vi "sub_new amplitude to array.vi"(6 "Index Row":i32, 7 "All Random Array In":fxp<+/-,32,16>[][](array[numeric]), 8 "y offset new":i16=548 max=1000 step=1, 9 "x offset new":i16=548 max=1000 step=1, 10 "y amp. new":dbl=548.0 max=1000.0 step=1.0, 11 "x amp. new":dbl=548.0 max=1000.0 step=1.0) -> (2 "Every Random Array":fxp<+/-,32,16>[](array[numeric]), 3 "All Random Array Out":fxp<+/-,32,16>[][](array[numeric]) format="%.42g")   [LabVIEW 2015]
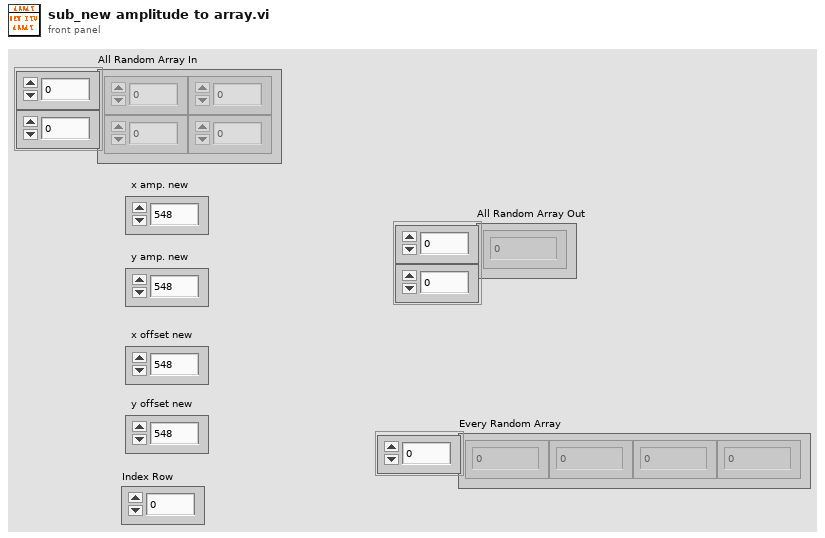
[diagram p1: front panel]
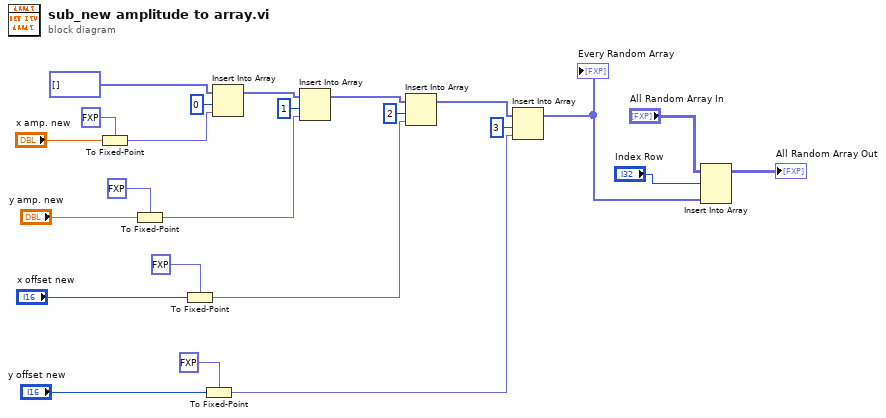
[diagram p0: block diagram]
diagram:
  n1 = To Fixed-Point(fixed-point type=fxp<+/-,32,16> 0.0 ("定点类型"), number="x amp. new") -> (fixed-point=w8:fxp<+/-,32,16>)
  n2 = To Fixed-Point(fixed-point type=fxp<+/-,32,16> 0.0 ("定点类型"), number="y amp. new") -> (fixed-point=w7:fxp<+/-,32,16>)
  n3 = To Fixed-Point(fixed-point type=fxp<+/-,32,16> 0.0 ("定点类型"), number="x offset new") -> (fixed-point=w6:fxp<+/-,32,16>)
  n4 = To Fixed-Point(fixed-point type=fxp<+/-,32,16> 0.0 ("定点类型"), number="y offset new") -> (fixed-point=w5:fxp<+/-,32,16>)
  n5 = Insert Into Array(array=fxp<+/-,32,16>[] [] ("数组"), index=0 ("索引"), new element=w8) -> (w16:fxp<+/-,32,16>[])
  n6 = Insert Into Array(array=w16, index=1 ("索引"), new element=w7) -> (w15:fxp<+/-,32,16>[])
  n7 = Insert Into Array(array=w15, index=2 ("索引"), new element=w6) -> (w14:fxp<+/-,32,16>[])
  n8 = Insert Into Array(array=w14, index=3 ("索引"), new element=w5) -> (w12:fxp<+/-,32,16>[])
  "Every Random Array" <- w12
  n9 = Insert Into Array(array="All Random Array In", index (row)="Index Row", new element=w12) -> (→"All Random Array Out":fxp<+/-,32,16>[][])  [unwired: 1 in]
